vi "batch action return immediately.vi"() -> ()   [LabVIEW 2013]
uses:
  standard tasks/batch task/reporting type.ctl
  result/result.lvclass/result.ctl
  result/get data.vi
  result/get error.vi
  result/get data ID.vi
  dispatcher/thread pool.lvclass
  standard reporters/event reporter/event reporter.lvclass
  result/result.lvclass
  standard tasks/batch task/batch task.lvclass
  standard action/wait action/wait action.lvclass
panel:
  out "result names":string[](array[string])
  out "event times":u32[](array[numeric])
  out "iteration":i32
  out "errors":errorcluster[](array[cluster])
  out "data":variant[](array[variant])
  out "Time":u32
  out "error out":errorcluster
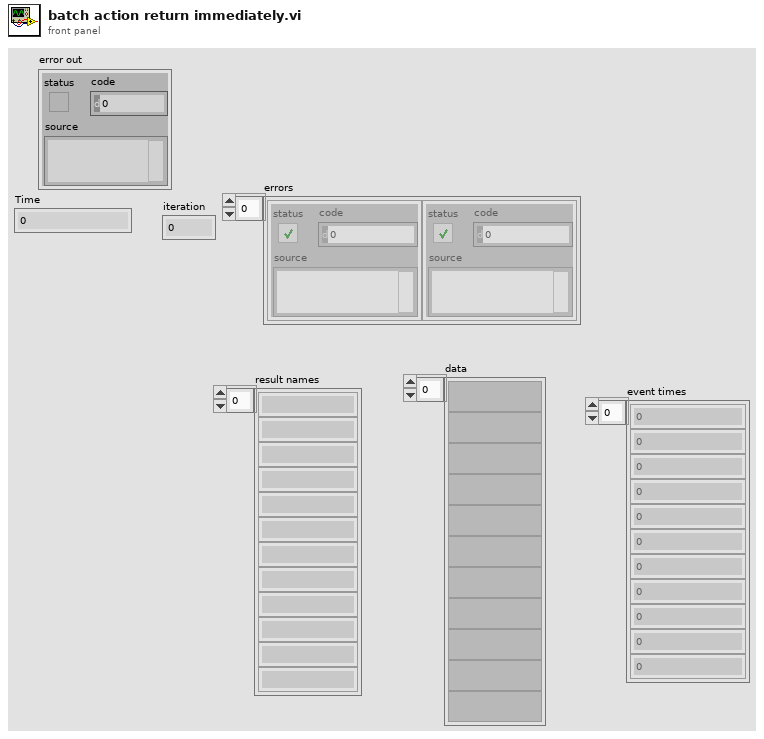
[diagram p1: front panel]
types:
  T1 = typedef "batch task.lvclass/reporting type.ctl" = enum16{"return immediately", "wait on all"}
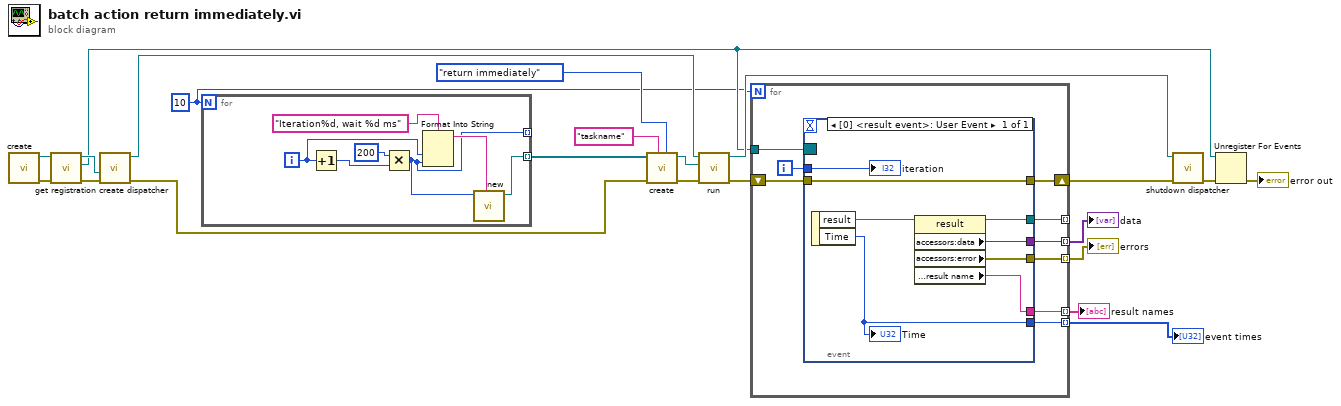
[diagram p0: block diagram]
diagram:
  w3 = 10 ("dimension size")
  n1 = call "create.vi"() -> ("error out"=w19:errorcluster, "event reporter out"=w20:refnum<class "event reporter.lvclass">)  [unwired: 10 in]
  n2 = call "get registration.vi"("error in"=w19, "event reporter in"=w20) -> ("error out"=w17:errorcluster, "result registration"=w9:refnum<event-registration>, "event reporter out"=w18:refnum<class "event reporter.lvclass">)  [unwired: 7 in]
  n3 = call "create dispatcher.vi"("error in"=w17, "default reporter"=w18) -> ("error out"=w1:errorcluster, "dispatcher"=w21:refnum<data-value>)  [unwired: 8 in]
  n4 = for {
    N: w3 -> [_]
    tunnel: [w22] -> _ mode=indexing
    tunnel: [w24] -> w4 mode=indexing
    i -> [w28]
    n5 = Increment(x=w28) -> (x+1=w27:i32)
    n6 = Multiply(x=200, y=w27) -> (x*y=w22:i32)
    n7 = Format Into String(format string="Iteration%d, wait %d ms", w28, w22) -> (resulting string=w23:string)  [unwired: 2 in, 1 out]
    n8 = call "new.vi"("ID"=w23, "timer"=w22) -> ("wait action out"=w24:refnum<class "wait action.lvclass">)  [unwired: 9 in]
  }
  n9 = call "create.vi"("reporting type"=reporting_type."return immediately", "ID"="taskname", "tasks"=w4) -> ("batch task out"=w11:refnum<class "batch task.lvclass">)  [unwired: 8 in]
  n10 = call "run.vi"("error in"=w1, "task"=w11, "dispatcher"=w21) -> ("error out"=w12:errorcluster, "dispatcher out"=w16:refnum<data-value>)  [unwired: 7 in]
  n11 = for {
    N: w3 -> [_]
    tunnel: w9 -> [w37]
    shift-right: [w36] -> w13
    shift-left: w12 -> [w35]
    tunnel: [w34] -> w8 mode=indexing
    tunnel: [w33] -> w7 mode=indexing
    tunnel: [w32] -> _ mode=indexing
    tunnel: [w30] -> w6 mode=indexing
    tunnel: [w29] -> w2 mode=indexing
    i -> [w31]
    n12 = event shown="[0] <result event>: User Event" {
      selector: w37 -> [_]
      dyn-events: _ -> [_]
      timeout: _ -> [_]
      tunnel: [w45] -> w36
      tunnel: w35 -> [w45]
      tunnel: [w43] -> w34
      tunnel: [w42] -> w33
      tunnel: [w41] -> w32
      tunnel: w31 -> [w40]
      tunnel: [w39] -> w30
      tunnel: [w38] -> w29
      event User Event {
        n13 = event-data() -> ("result"=w44:refnum<class "result.lvclass">, "Time"=w39:u32)  [unwired: 1 in]
        "Time" <- w39
        n14 = property class="result"(reference=w44) -> (reference out=w41:refnum<class "result.lvclass">, "accessors:data"=w43:variant, "accessors:error"=w42:errorcluster, "accessors:result name"=w38:string)  [unwired: 1 in, 1 out]
        "iteration" <- w40
      }
    }
  }
  "data" <- w8
  "errors" <- w7
  "event times" <- w6
  "result names" <- w2
  n15 = call "shutdown dispatcher.vi"("error in"=w13, "dispatcher"=w16) -> ("error out"=w15:errorcluster)  [unwired: 9 in]
  n16 = Unregister For Events(event registration refnum=w9, error in=w15) -> (error out=→"error out":errorcluster)
